vi "Put-Ball_Lite.vi"(6 "輸出顏色-位置":T1(array[cluster]), 8 "Error In":errorcluster, 11 "HiTechnicColorSensorV2 Ref In":cluster{"I2C Ref Out":T2}) -> (0 "Error Out":errorcluster, 3 "HiTechnicColorSensorV2 Ref Out":cluster{"I2C Ref Out":T2}, 4 "輸出顏色-位置":T1(array[cluster]))   [LabVIEW 2019]
uses:
  <vilib>/myRIO/Instrument Drivers/Onboard IO/I2C/typedefs/I2C Reference.ctl
  <vilib>/myRIO/Common/Instrument Driver Framework/Utilities/typedefs/myRIO Generic Hardware Reference.ctl
  <vilib>/myRIO/Common/Instrument Driver Framework/Utilities/typedefs/Hardware Version Enum.ctl
  <vilib>/myRIO/Common/Instrument Driver Framework/Utilities/typedefs/myRIO v1.0 Reference.ctl
  <vilib>/myRIO/Common/Instrument Driver Framework/Utilities/typedefs/Generic FPGA Reference.ctl
  <vilib>/myRIO/Common/Instrument Driver Framework/myRIO v1.0/I2C/typedefs/I2C Channels Enum.ctl
  <vilib>/myRIO/Instrument Drivers/Onboard IO/I2C/typedefs/I2C Configuration.ctl
  <vilib>/myRIO/Instrument Drivers/Onboard IO/I2C/typedefs/I2C Transfer Rate.ctl
  <vilib>/myRIO/Instrument Drivers/Onboard IO/I2C/I2C.lvlib
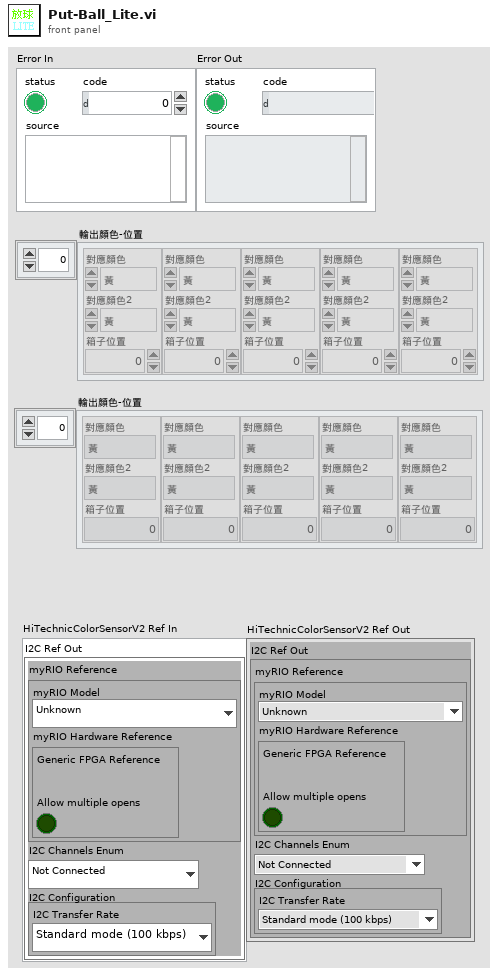
[diagram p1: front panel]
types:
  T1 = cluster{"對應顏色":enum16{"黃", "紅", "綠", "藍", "黑", "無"}, "對應顏色2":enum16{"黃", "紅", "綠", "藍", "黑", "無"}, "箱子位置":i32}[]
  T2 = typedef "I2C.lvlib/I2C Reference.ctl" = cluster{"myRIO Reference":T3, "I2C Channels Enum":T7, "I2C Configuration":T8}
  T3 = typedef "myRIO Generic Hardware Reference.ctl" = cluster{"myRIO Model":T4, "myRIO Hardware Reference":T5}
  T4 = typedef "Hardware Version Enum.ctl" = enum16{"Unknown", "myRIO-1900", "myRIO-1950", "roboRIO", "NI ELVIS RIO CM", "ELVIS III"}
  T5 = typedef "myRIO v1.0 Reference.ctl" = cluster{"Generic FPGA Reference":T6, "Allow multiple opens":bool}
  T6 = typedef "Generic FPGA Reference.ctl" = refnum<k20>
  T7 = typedef "I2C Channels Enum.ctl" = enum16{"Not Connected", "A/I2C", "B/I2C", "I2C/I2C"}
  T8 = typedef "I2C.lvlib/I2C Configuration.ctl" = cluster{"I2C Transfer Rate":T9}
  T9 = typedef "I2C.lvlib/I2C Transfer Rate.ctl" = enum16{"Standard mode (100 kbps)", "Fast mode (400 kbps)"}
  T10 = enum16{"前", "後", "オ", "右", "無", "0", "1", "2", "3", "4", "5", "6", "7"}
  T11 = cluster{"執行放球?":bool, "執行補值、校正?":bool, "當前位置":i32, "目標位置":i32}
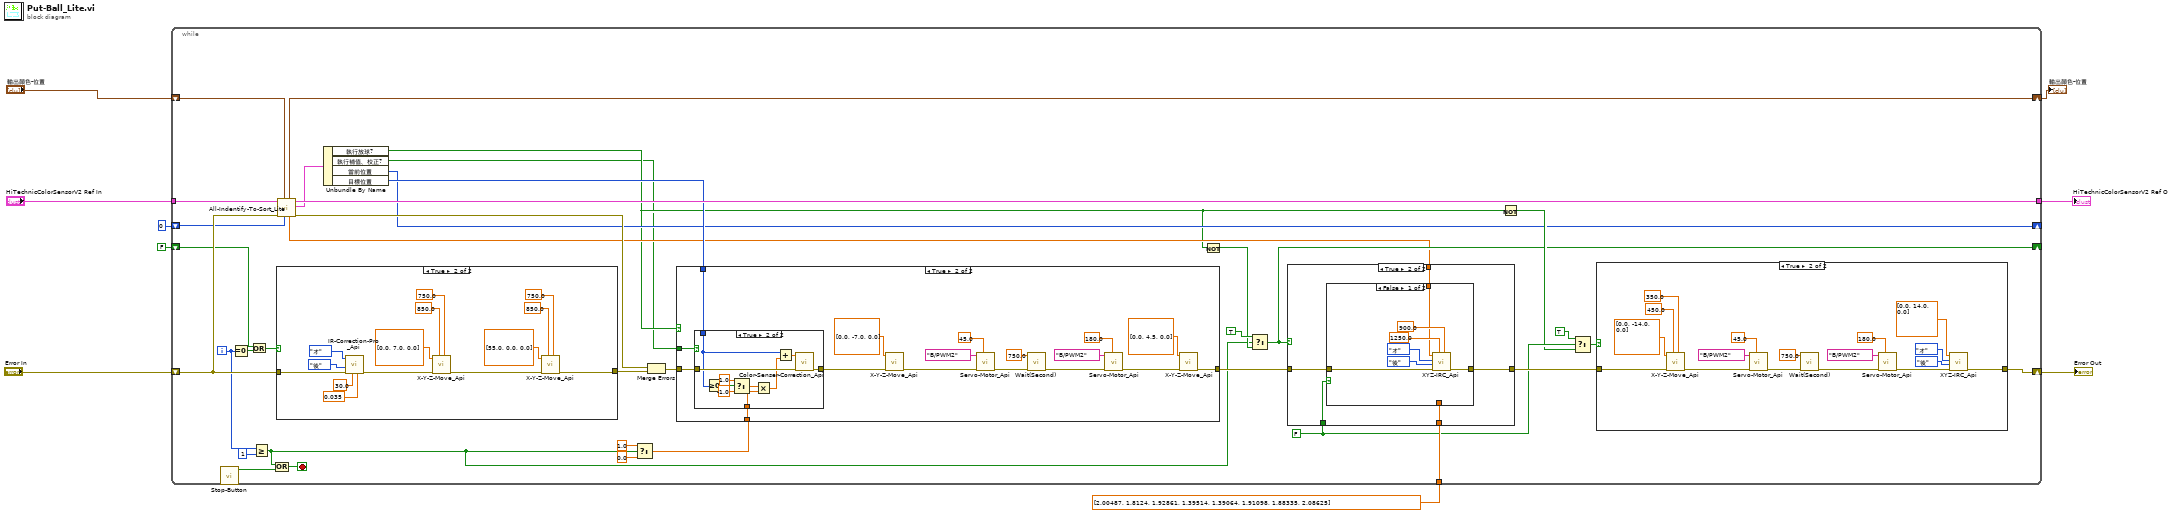
[diagram p0: block diagram]
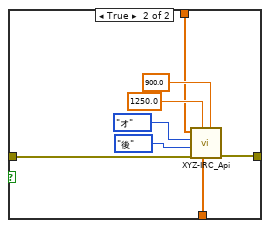
[diagram p5: hidden frame]
diagram:
  n1 = while {
    tunnel: dbl[] [2.00487, 1.8124, 1.92861, 1.39514, 1.39064, 1.91098, 1.88335, 2.08625] ("目標電壓") -> [w38]
    shift-right: [w42] -> w6
    shift-left: "Error In" -> [w46]
    tunnel: "HiTechnicColorSensorV2 Ref In" -> [w45]
    tunnel: [w44] -> w7
    shift-right: [w12] -> w4
    shift-left: "輸出顏色-位置" -> [w36]
    shift-right: [w21] -> _
    shift-left: 0 ("當前位置") -> [w35]
    shift-right: [w19] -> _
    shift-left: FALSE -> [w25]
    i -> [w32]
    stop <- w34 stop-if-true
    w29 = FALSE ("回起始點?")
    n2 = call "Stop-Button.vi"() -> ("顯示按下?"=w33:bool)  [unwired: 10 in, 1 out]
    n3 = Equal To 0?(x=w32) -> (x = 0?=w26:bool)
    n4 = Or(x=w25, y=w26) -> (x .or. y?=w24:bool)
    n5 = Greater Or Equal?(x=w32, y=1) -> (x >= y?=w14:bool)
    n6 = Compound Arithmetic op=OR(w14, w33) -> (w34:bool)
    n7 = case shown="True" w24 {
      tunnel: w46 -> [w47 w54]
      tunnel: [w47 w48] -> w41
      frame False {
      }
      frame True {
        n8 = call "IR-Correction-Pro_Api.vi"("ExitRange"=0.035, "精準度"=30.0, "Error In"=w54, "副邊校正"=T10."後", "主編校正"=enum16{"前", "後", "オ", "右", "無"}."オ") -> ("Error Out"=w53:errorcluster)  [unwired: 6 in]
        n9 = call "X-Y-Z-Move_Api.vi"("加速度"=750.0, "最高速"=850.0, "Error In"=w53, "X-Y-Z移動"=dbl[] [0.0, 7.0, 0.0]) -> ("Error Out"=w49:errorcluster)  [unwired: 6 in, 1 out]
        n10 = call "X-Y-Z-Move_Api.vi"("加速度"=750.0, "最高速"=850.0, "Error In"=w49, "X-Y-Z移動"=dbl[] [55.0, 0.0, 0.0]) -> ("Error Out"=w48:errorcluster)  [unwired: 6 in, 1 out]
      }
    }
    n11 = call "All-Indentify-To-Sort_Lite.vi"("當前位置"=w35, "輸出顏色-位置"=w36, "Error In"=w46, "HiTechnicColorSensorV2 Ref In"=w45) -> ("Error Out"=w43:errorcluster, "判斷結果"=w23:T11, "HiTechnicColorSensorV2 Ref Out"=w44:cluster{"I2C Ref Out":T2}, "離家數值"=w13:dbl[], "輸出顏色-位置 2"=w12:T1)  [unwired: 3 in]
    n12 = Unbundle By Name(w23) -> ("執行放球?"=w11:bool, "執行補值、校正?"=w10:bool, "當前位置"=w21:i32, "目標位置"=w22:i32)
    n13 = Select(t=1.0, s=w14, f=0.0) -> (s? t:f=w17:dbl)
    n14 = Merge Errors(w43, w41) -> (w40:errorcluster)
    n15 = case shown="True" w11 {
      tunnel: w40 -> [w101 w105]
      tunnel: [w101 w106] -> w39
      tunnel: w22 -> [_ w104]
      tunnel: w17 -> [_ w103]
      tunnel: w10 -> [_ w102]
      frame False {
      }
      frame True {
        n16 = case shown="True" w102 {
          tunnel: [w119 w129] -> w118
          tunnel: w105 -> [w119 w128]
          tunnel: w104 -> [_ w126]
          tunnel: w103 -> [_ w121]
          frame False {
          }
          frame True {
            n17 = Greater Or Equal To 0?(x=w126) -> (x >= 0?=w125:bool)
            n18 = Select(t=1.0, s=w125, f=-1.0) -> (s? t:f=w122:dbl)
            n19 = Multiply(x=w122, y=w121) -> (x*y=w120:dbl)
            n20 = Add(x=w126, y=w120) -> (x+y=w127:dbl)
            n21 = call "Color-Senser-Correction_Api.vi"("Error In"=w128, "接收位置"=w127) -> ("Error Out"=w129:errorcluster)  [unwired: 9 in]
          }
        }
        n22 = call "X-Y-Z-Move_Api.vi"("Error In"=w118, "X-Y-Z移動"=dbl[] [0.0, -7.0, 0.0]) -> ("Error Out"=w116:errorcluster)  [unwired: 8 in, 1 out]
        n23 = call "Servo-Motor_Api.vi"("角度"=45.0, "Error In"=w116, "伺服馬達角位"=tag "B/PWM2") -> ("Error Out"=w113:errorcluster)  [unwired: 8 in]
        n24 = call "Wait(Second).vi"("Error In"=w113, "等待秒數(3000毫秒)"=750.0) -> ("Error Out"=w109:errorcluster)  [unwired: 9 in]
        n25 = call "Servo-Motor_Api.vi"("角度"=180.0, "Error In"=w109, "伺服馬達角位"=tag "B/PWM2") -> ("Error Out"=w107:errorcluster)  [unwired: 8 in]
        n26 = call "X-Y-Z-Move_Api.vi"("Error In"=w107, "X-Y-Z移動"=dbl[] [0.0, 4.5, 0.0]) -> ("Error Out"=w106:errorcluster)  [unwired: 8 in, 1 out]
      }
    }
    n27 = Not(x=w11) -> (.not. x?=w18:bool)
    n28 = Select(t=TRUE, s=w14, f=w18) -> (s? t:f=w19:bool)
    n29 = case shown="True" w19 {
      tunnel: w39 -> [w80 w85]
      tunnel: [w80 w82] -> w37
      tunnel: w29 -> [_ w84]
      tunnel: w38 -> [_ w83]
      tunnel: w13 -> [_ w81]
      frame False {
      }
      frame True {
        n30 = case shown="False" w84 {
          tunnel: w85 -> [w91 w99]
          tunnel: [w90 w98] -> w82
          tunnel: w83 -> [_ w96]
          tunnel: w81 -> [w86 w93]
          frame False {
            n31 = call "XYZ-IRC_Api.vi"("加速度"=900.0, "最高速"=1250.0, "Error"=w91, "副邊校正"=T10."後", "主編校正"=enum16{"前", "後", "オ", "右", "無"}."オ", "X-Y-Z移動"=w86) -> ("Error Out"=w90:errorcluster)  [unwired: 5 in]
          }
          frame True {
            n32 = call "XYZ-IRC_Api.vi"("加速度"=900.0, "目標電壓"=w96, "最高速"=1250.0, "Error"=w99, "副邊校正"=T10."後", "主編校正"=enum16{"前", "後", "オ", "右", "無"}."オ", "X-Y-Z移動"=w93) -> ("Error Out"=w98:errorcluster)  [unwired: 4 in]
          }
        }
      }
    }
    n33 = Not(x=w11) -> (.not. x?=w27:bool)
    n34 = Select(t=TRUE, s=w29, f=w27) -> (s? t:f=w30:bool)
    n35 = case shown="True" w30 {
      tunnel: [w62 w63] -> w42
      tunnel: w37 -> [w62 w78]
      frame False {
      }
      frame True {
        n36 = call "X-Y-Z-Move_Api.vi"("加速度"=350.0, "最高速"=450.0, "Error In"=w78, "X-Y-Z移動"=dbl[] [0.0, -14.0, 0.0]) -> ("Error Out"=w75:errorcluster)  [unwired: 6 in, 1 out]
        n37 = call "Servo-Motor_Api.vi"("角度"=45.0, "Error In"=w75, "伺服馬達角位"=tag "B/PWM2") -> ("Error Out"=w72:errorcluster)  [unwired: 8 in]
        n38 = call "Wait(Second).vi"("Error In"=w72, "等待秒數(3000毫秒)"=750.0) -> ("Error Out"=w68:errorcluster)  [unwired: 9 in]
        n39 = call "Servo-Motor_Api.vi"("角度"=180.0, "Error In"=w68, "伺服馬達角位"=tag "B/PWM2") -> ("Error Out"=w65:errorcluster)  [unwired: 8 in]
        n40 = call "XYZ-IRC_Api.vi"("Error"=w65, "副邊校正"=T10."後", "主編校正"=enum16{"前", "後", "オ", "右", "無"}."オ", "X-Y-Z移動"=dbl[] [0.0, 14.0, 0.0]) -> ("Error Out"=w63:errorcluster)  [unwired: 7 in]
      }
    }
  }
  "HiTechnicColorSensorV2 Ref Out" <- w7
  "Error Out" <- w6
  "輸出顏色-位置" <- w4
